vi "readingStatusID.vi"(8 "error in (no error)":errorcluster, 11 "ElectrometerReadingStatus in":refnum<class "ElectrometerReadingStatus.lvclass">) -> (0 "error out":errorcluster, 2 "Reading?":bool, 3 "ElectrometerReadingStatus out":refnum<class "ElectrometerReadingStatus.lvclass">)   [LabVIEW 2016, in "ElectrometerReadingStatus.lvclass"]
uses:
  ElectrometerReadingStatus.lvclass
  ElectrometerReadingVar.vi
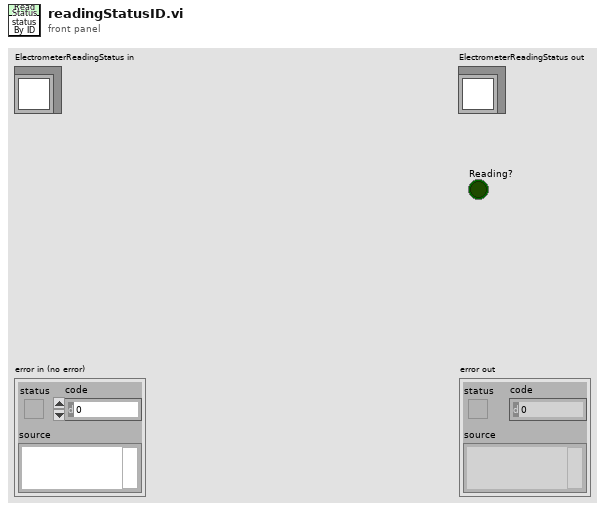
[diagram p1: front panel]
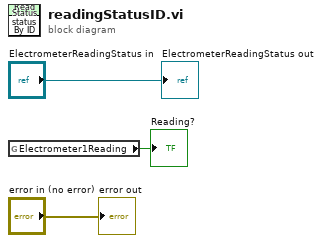
[diagram p0: block diagram]
diagram:
  n1 = global read "ElectrometerReadingVar.vi" "Electrometer1Reading"() -> (→"Reading?":bool)
  "error out" <- "error in (no error)"
  "ElectrometerReadingStatus out" <- "ElectrometerReadingStatus in"
